vi "Activ ALRB.vi"(10 "Ack":bool[](array[boolean]), 11 "ALR":bool[](array[boolean])) -> (1 "A alr":bool[](array[boolean]), 2 "R alr":bool[](array[boolean]), 3 "T alr":bool[](array[boolean]))   [LabVIEW 2019, in "Alarms.lvlib"]
uses:
  Alarms.lvlib
  Trigers/Triggers.lvlib
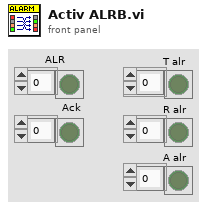
[diagram p1: front panel]
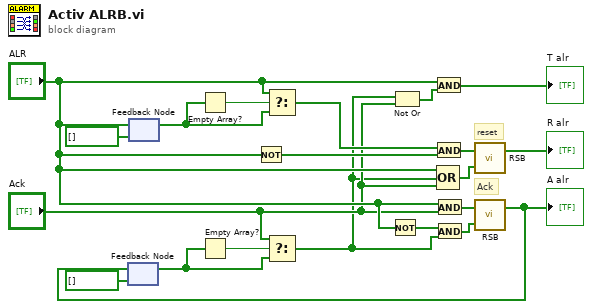
[diagram p0: block diagram]
diagram:
  # "Ack"
  # "reset"
  n1 = feedback #1(bool[] [] ("Q")) -> (w17:bool[])
  n2 = feedback #2(bool[] [] ("ALR")) -> (w16:bool[])
  n3 = feedback-in #2("ALR") -> ()
  n4 = Empty Array?(array=w16) -> (empty?=w15:bool)
  n5 = Empty Array?(array=w17) -> (empty?=w18:bool)
  n6 = Not(x="ALR") -> (.not. x?=w9:bool[])
  n7 = Select(t="ALR", s=w15, f=w16) -> (s? t:f=w8:bool[])
  n8 = Select(t="Ack", s=w18, f=w17) -> (s? t:f=w3:bool[])
  n9 = Not(x="ALR") -> (.not. x?=w10:bool[])
  n10 = Not Or(1:"Ack", 2:w3) -> (0:w7:bool[])
  n11 = And(x="ALR", y=w7) -> (x .and. y?=→"T alr":bool[])
  n12 = And(x=w8, y=w9) -> (x .and. y?=w12:bool[])
  n13 = And(x="ALR", y="Ack") -> (x .and. y?=w20:bool[])
  n14 = And(x=w10, y=w3) -> (x .and. y?=w13:bool[])
  n15 = Compound Arithmetic op=OR("ALR", w3, "Ack") -> (w14:bool[])
  n16 = call "RSB.vi"("R"=w14, "S"=w12) -> ("Q"=→"R alr":bool[])  [unwired: 1 out]
  n17 = call "RSB.vi"("R"=w13, "S"=w20) -> ("Q"=w19:bool[])  [unwired: 1 out]
  "A alr" <- w19
  n18 = feedback-in #1(w19) -> ()
